vi "scan string for tokens.vi"(10 "operators":string[](array[string]), 11 "input string":string) -> (2 "token string":string, 3 "string out":string)   [LabVIEW 2024, in "controls manager.lvlib"]
uses:
  controls manager.lvlib
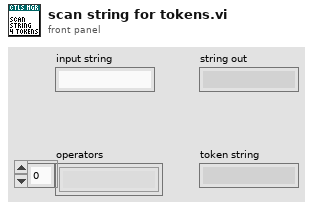
[diagram p1: front panel]
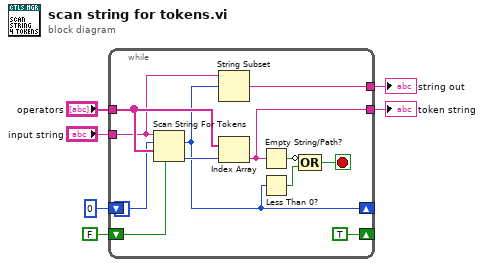
[diagram p0: block diagram]
diagram:
  n1 = while {
    shift-right: [w9] -> _
    shift-left: 0 -> [w10]
    tunnel: "input string" -> [w8]
    shift-right: [TRUE] -> _
    shift-left: FALSE -> [w18]
    tunnel: "operators" -> [w16]
    tunnel: [w12] -> w6
    tunnel: [w7] -> w1
    stop <- w13 stop-if-true
    n2 = Scan String For Tokens(4:w18, 7:w16, 8:w10, 9:w8) -> (0:w15:i32, 2:w9:i32)  [unwired: 2 in, 2 out]
    n3 = String Subset(string=w8, offset (0)=w9) -> (substring=w7:string)  [unwired: 1 in]
    n4 = Index Array(array=w16, index=w15) -> (element=w12:string)
    n5 = Empty String/Path?(string/path=w12) -> (empty?=w14:bool)
    n6 = Less Than 0?(x=w9) -> (x < 0?=w11:bool)
    n7 = Compound Arithmetic op=OR(invert w14, w11) -> (w13:bool)
  }
  "token string" <- w6
  "string out" <- w1
